vi "Design request string.vi"(8 "error in (no error)":errorcluster, 11 "DesignRequest":T1) -> (0 "error out":errorcluster, 3 "String":string)   [LabVIEW 2012, in "Design Server.lvlib"]
uses:
  Design Server.lvlib
  Design Request.ctl
  Variable cluster.ctl
panel:
  in  "NewYear2012":timestamp=timestamp(3408238800 s since 1904-01-01)
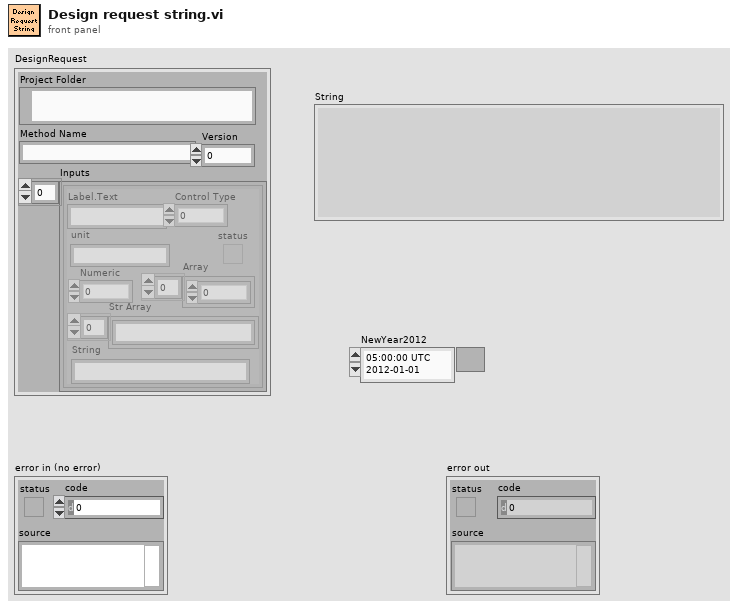
[diagram p1: front panel]
types:
  T1 = typedef "Design Server.lvlib/Design Request.ctl" = cluster{"Project Folder":path, "Method Name":string, "Inputs":T2, "Version":i32}
  T2 = typedef "Design Server.lvlib/Variable cluster.ctl" = cluster{"Label.Text":string, "Control Type":u32, "Numeric":dbl, "Array":dbl[], "status":bool, "Str Array":string[], "String":string, "unit":string}[]
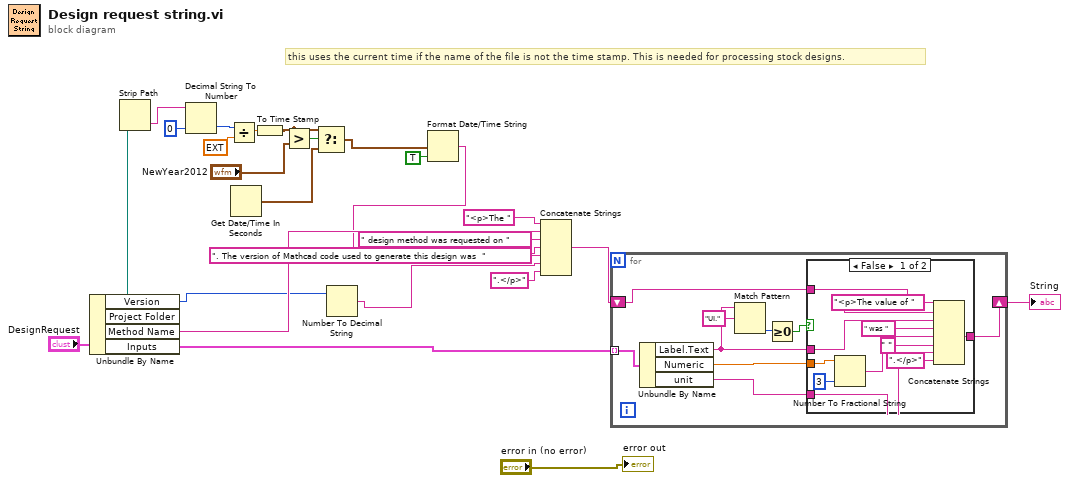
[diagram p0: block diagram]
diagram:
  # "this uses the current time if the name of the file is not the time stamp. This is needed for processing stock designs."
  n1 = Unbundle By Name("DesignRequest") -> ("Version"=w2:i32, "Project Folder"=w17:path, "Method Name"=w22:string, "Inputs"=w25:T2)
  n2 = Strip Path(path=w17) -> (name=w12:string)  [unwired: 1 out]
  n3 = Decimal String To Number(string=w12, default (0L)=i64 0 ("default (0 I32)")) -> (number=w14:i64)  [unwired: 1 in, 1 out]
  n4 = Divide(x=w14, y=ext 100.0) -> (x/y=w15:ext)
  n5 = Get Date/Time In Seconds() -> (seconds since 1Jan1904=w6:timestamp)
  n6 = To Time Stamp(1:w15) -> (0:w7:timestamp)
  n7 = Greater?(x=w7, y="NewYear2012") -> (0:w8:bool)
  n8 = Select(t=w7, s=w8, f=w6) -> (s? t:f=w5:timestamp)
  n9 = Number To Decimal String(number=w2) -> (decimal integer string=w1:string)  [unwired: 1 in]
  n10 = Format Date/Time String(seconds (now)=w5, UTC format=TRUE) -> (date/time string=w10:string)  [unwired: 1 in]
  n11 = Concatenate Strings("<p>The ", w22, " design method was requested on " ("string"), w10, ". The version of Mathcad code used to generate this design was  " ("string"), w1, ".</p>" ("string")) -> (w20:string)
  n12 = for {
    tunnel: w25 -> [w34] mode=indexing
    shift-right: [w27] -> w23
    shift-left: w20 -> [w26]
    n13 = Unbundle By Name(w34) -> ("Label.Text"=w31:string, "Numeric"=w33:dbl, "unit"=w32:string)
    n14 = Match Pattern(string=w31, regular expression="UI.") -> (offset past match=w29:i32)  [unwired: 1 in, 3 out]
    n15 = Greater Or Equal To 0?(x=w29) -> (x >= 0?=w28:bool)
    n16 = case shown="False" w28 {
      tunnel: w33 -> [w45 _]
      tunnel: w32 -> [w40 _]
      tunnel: w31 -> [w38 _]
      tunnel: [w37 w46] -> w27
      tunnel: w26 -> [w36 w46]
      frame False {
        n17 = Number To Fractional String(number=w45, precision (6)=i16 3) -> (F-format string=w42:string)  [unwired: 2 in]
        n18 = Concatenate Strings(w36, "<p>The value of ", w38, " was " ("string"), w42, " " ("string"), w40, ".</p>" ("string")) -> (w37:string)
      }
      frame True {
      }
    }
  }
  "String" <- w23
  "error out" <- "error in (no error)"
